vi "Tests.vi"() -> ()   [LabVIEW 2024]
uses:
  TesterModule/TesterModule.lvclass
  C:/DevOps/CORTEX/JQMH/JQMHCore/Module/JQMHModule.lvclass
  JQMHCore/Module/JQMHModule.lvclass
panel:
  in  "stop":bool
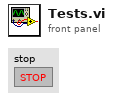
[diagram p1: front panel]
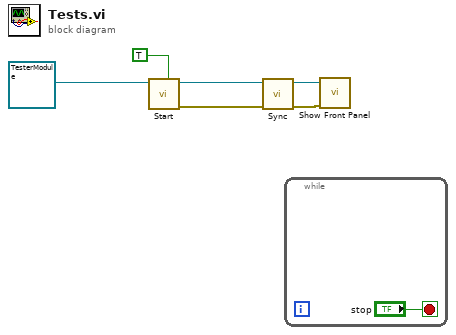
[diagram p0: block diagram]
diagram:
  n1 = call "Start.vi"("Autoshutdown? (T)"=TRUE, "JQMHCore in"=refnum<class "TesterModule.lvclass"> refnum ("TesterModule.lvclass")) -> ("error out"=w5:errorcluster, "JQMHCore out"=w6:refnum<class "JQMHModule.lvclass">)  [unwired: 8 in]
  n2 = call "Sync.vi"("error in (no error)"=w5, "JQMHCore in"=w6) -> ("error out"=w2:errorcluster, "JQMHCore out"=w3:refnum<class "JQMHModule.lvclass">)  [unwired: 8 in]
  n3 = while {
    stop <- "stop" stop-if-true
  }
  n4 = call "Show Front Panel.vi"("error in (no error)"=w2, "JQMHCore in"=w3) -> ()  [unwired: 8 in, 2 out]
